vi "sendmail.vi"(6 "error in":errorcluster, 7 "dry_run":bool, 9 "message":string caption="Message", 10 "title":string, 11 "address_array":string[](array[string])=["", ""]) -> (2 "full_title":string, 3 "full_address":string, 4 "error out":errorcluster)   [LabVIEW 2019]
panel:
  out "date_time":timestamp format="%<%Y-%m-%d %H:%M:%S>T"
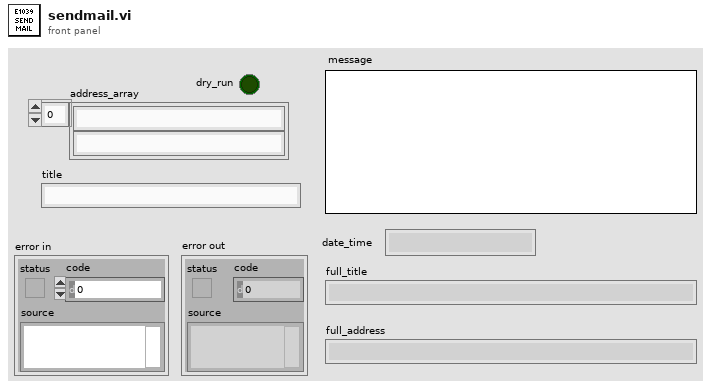
[diagram p1: front panel]
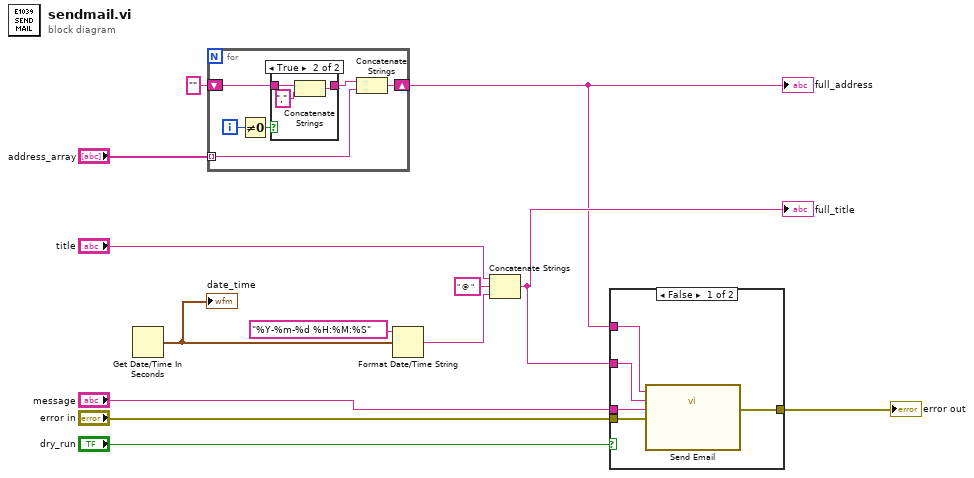
[diagram p0: block diagram]
diagram:
  n1 = Get Date/Time In Seconds() -> (seconds since 1Jan1904=w12:timestamp)
  "date_time" <- w12
  n2 = for {
    tunnel: "address_array" -> [w14] mode=indexing
    shift-right: [w16] -> w3
    shift-left: "" ("Recipients") -> [w17]
    i -> [w19]
    n3 = Not Equal To 0?(x=w19) -> (x != 0?=w18:bool)
    n4 = case shown="True" w18 {
      tunnel: w17 -> [w20 w23]
      tunnel: [w20 w21] -> w15
      frame False {
      }
      frame True {
        n5 = Concatenate Strings(w23, "," ("string")) -> (w21:string)
      }
    }
    n6 = Concatenate Strings(w15, w14) -> (w16:string)
  }
  "full_address" <- w3
  n7 = Format Date/Time String(time format string (%c)="%Y-%m-%d %H:%M:%S", seconds (now)=w12) -> (date/time string=w9:string)  [unwired: 1 in]
  n8 = Concatenate Strings("title", " @ " ("string"), w9) -> (w4:string)
  "full_title" <- w4
  n9 = case shown="False" "dry_run" {
    tunnel: "error in" -> [w28 w29]
    tunnel: "message" -> [w27 _]
    tunnel: w4 -> [w26 _]
    tunnel: w3 -> [w25 _]
    tunnel: [w24 w29] -> w2
    frame False {
      n10 = call "Send Email"("error in"=w28, "Message"=w27, "Subject"=w26, "Recipients"=w25) -> ("error out"=w24:errorcluster)  [unwired: 7 in]
    }
    frame True {
    }
  }
  "error out" <- w2
